vi "reconstructAverageObject.vi"(9 "ctrlFactor":dbl, 10 "objRef":dbl[][](graph)) -> (1 "Frame count":dbl, 2 "objPro":dbl[][](graph), 3 "imgPro":dbl[][](graph), 11 "imgRaw":dbl[][](graph))   [LabVIEW 2012]
uses:
  <vilib>/Utility/error.llb/DialogType.ctl
panel:
  in  "Recon averaging":i32=1
  in  "Exposure Array (s)":dbl[](array[numeric])=[0.1]
  in  "Frames to average":i32=1
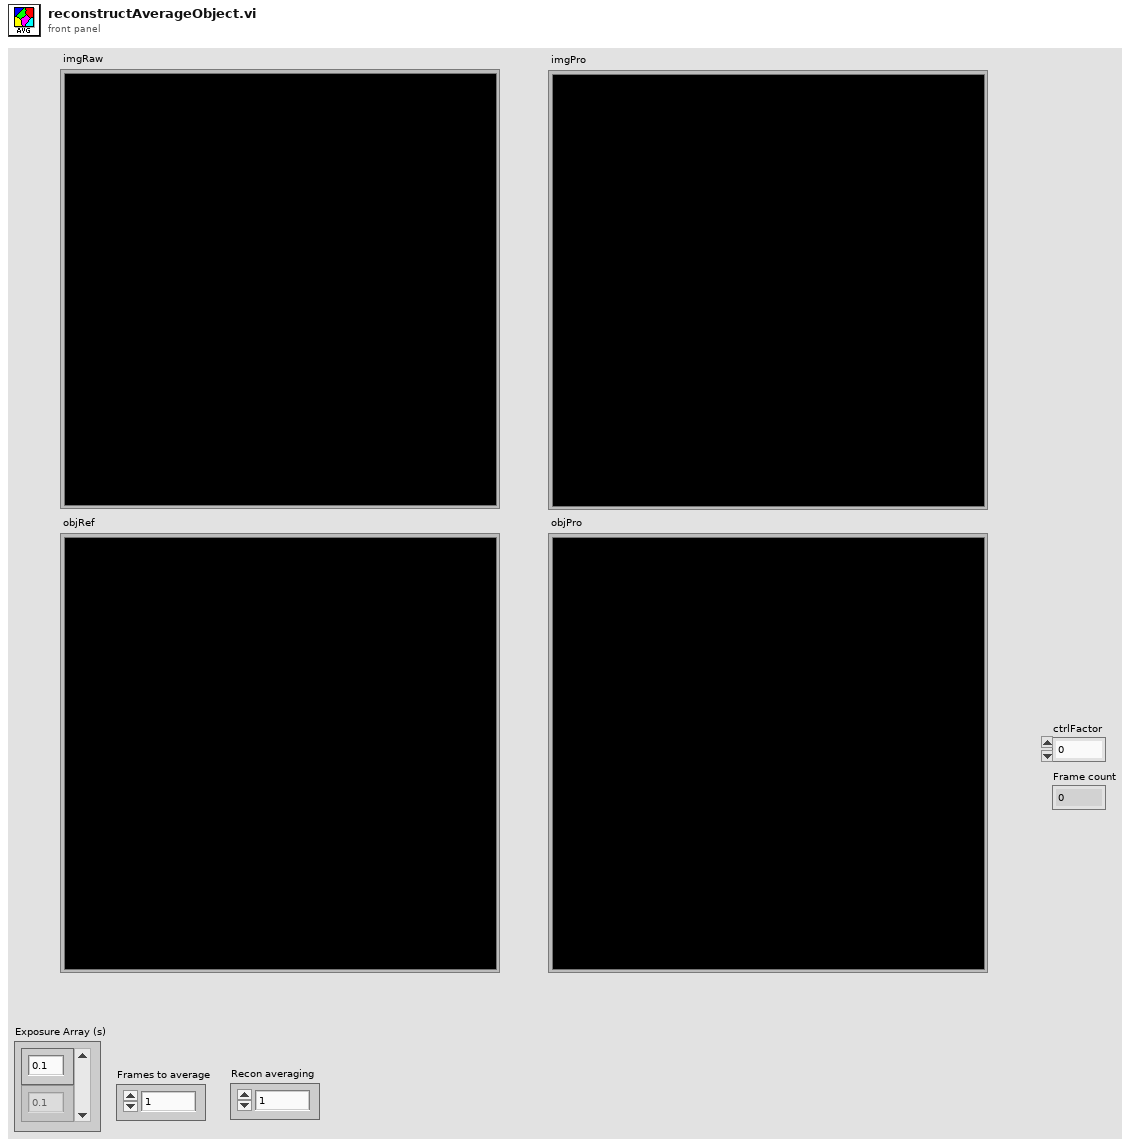
[diagram p1: front panel]
types:
  T1 = typedef "DialogType.ctl" = u16
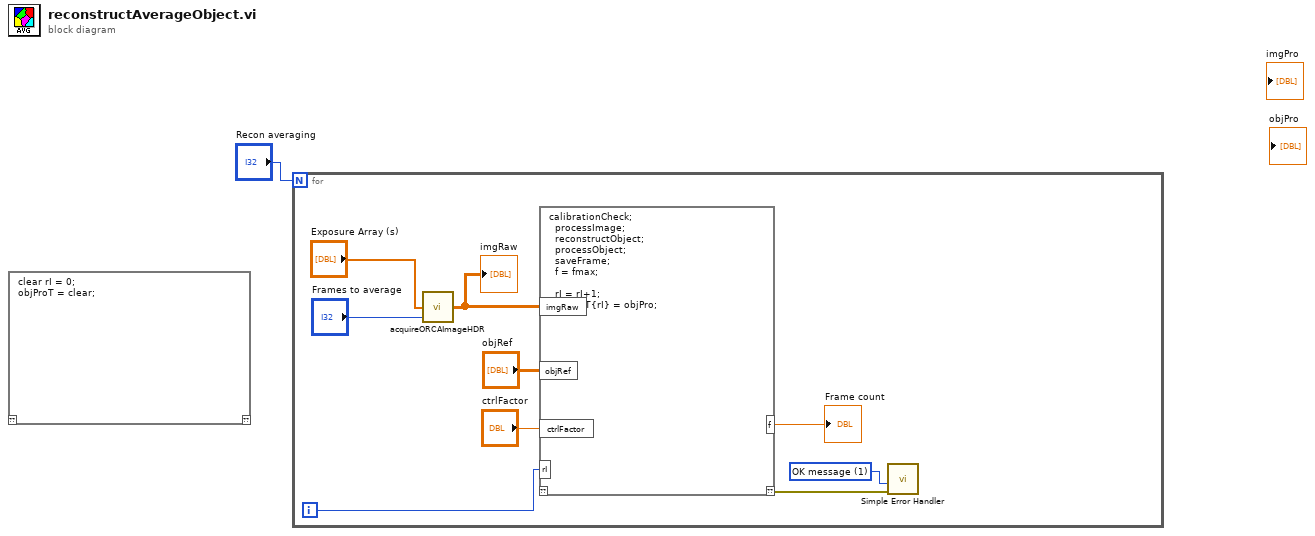
[diagram p0: block diagram]
diagram:
  n1 = script code="clear rI = 0;\nobjProT = clear;"() -> ()  [unwired: 1 in, 1 out]
  n2 = for {
    N: "Recon averaging" -> [_]
    i -> [w2]
    w6 = T1 1 items=["no dialog", "OK message", "continue or stop message", "OK message + warnings", "continue/stop + warnings"] ("type of dialog (OK msg:1)")
    n3 = call "acquireORCAImageHDR.vi"("Average"="Frames to average", "Exposure Array"="Exposure Array (s)") -> ("imgHDR"=w3:dbl[][])  [unwired: 1 in]
    "imgRaw" <- w3
    n4 = script code="calibrationCheck;\n  processImage;\n  reconstructObject;\n  processObject;\n  saveFrame;\n  f = fmax;\n\n  rI = rI+1;\n  objProT{rI} = objPro;"("imgRaw"=w3, "objRef"="objRef", "ctrlFactor"="ctrlFactor", "rI"=w2) -> ("??"=w7:errorcluster, "f"=→"Frame count":dbl)  [unwired: 1 in]
    n5 = call <vilib>:"Simple Error Handler.vi"("type of dialog (OK msg:1)"=w6, "error in (no error)"=w7) -> ()  [unwired: 3 in, 5 out]
  }
